vi "falpha.vi"(8 "fa":dbl, 9 "fbeta":dbl, 10 "Constants and System Parameters":T1) -> (2 "fapha":dbl)   [LabVIEW 2018]
uses:
  Constants and System Parameters.ctl
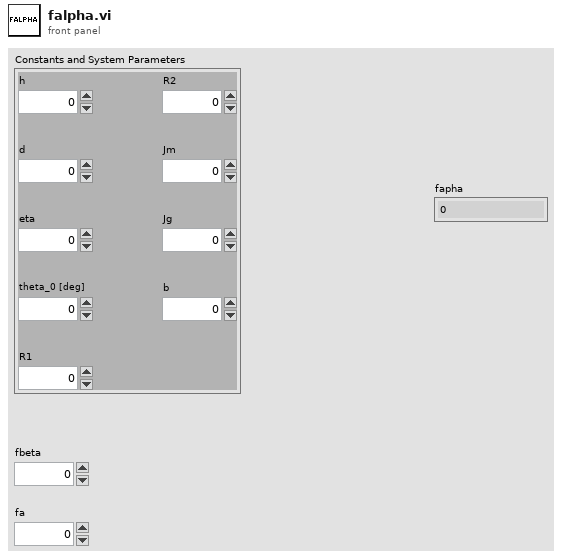
[diagram p1: front panel]
types:
  T1 = typedef "Constants and System Parameters.ctl" = cluster{"h":dbl, "d":dbl, "eta":dbl, "theta_0 [deg]":dbl, "R1":dbl, "R2":dbl, "Jm":dbl, "Jg":dbl, "b":dbl}
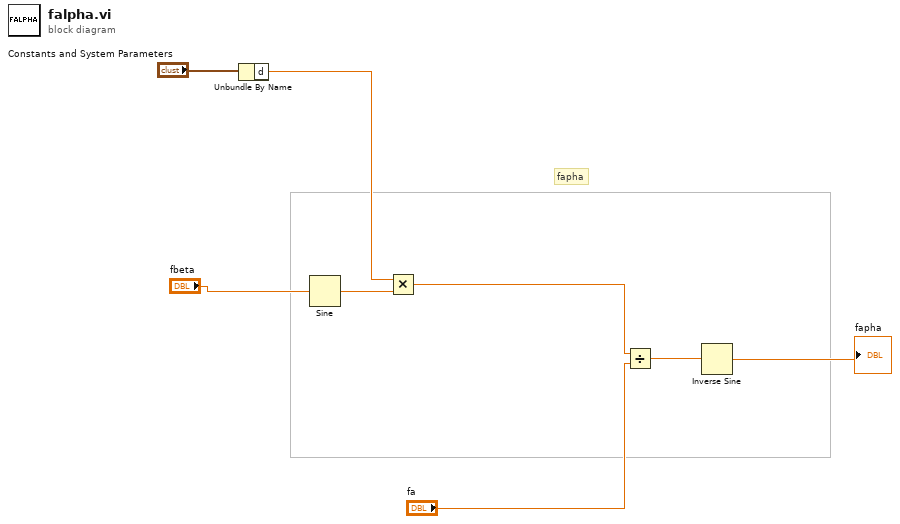
[diagram p0: block diagram]
diagram:
  # "fapha"
  n1 = Unbundle By Name("Constants and System Parameters") -> ("d"=w1:dbl)
  n2 = Sine(x="fbeta") -> (sin(x)=w8:dbl)
  n3 = Multiply(x=w1, y=w8) -> (x*y=w7:dbl)
  n4 = Divide(x=w7, y="fa") -> (x/y=w6:dbl)
  n5 = Inverse Sine(1:w6) -> (0:→"fapha":dbl)
